vi "Self Event.vi"(9 "Priority?":bool, 10 "Msg Strategy":refnum<class "Msg Strategy.lvclass">, 11 "Base Event in":refnum<class "Base Event.lvclass">) -> (3 "Base Event out":refnum<class "Base Event.lvclass">)   [LabVIEW 2021, in "jettl.lvlib" / "Base Event.lvlib" / "Base Event.lvclass"]
uses:
  Base Event.lvclass
  Msg Strategy/Msg Strategy.lvclass
  Base Event.lvclass/Base Event.ctl
  Self Event/Self Event.lvlib
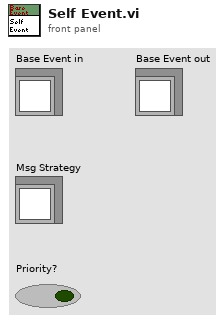
[diagram p1: front panel]
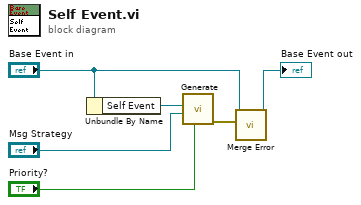
[diagram p0: block diagram]
diagram:
  n1 = Unbundle By Name("Base Event in") -> ("Self Event"=w5:refnum<data-value>)
  n2 = call "Generate.vi"("Priority?"="Priority?", "Msg Strategy"="Msg Strategy", "Self Event"=w5) -> ("error out"=w6:errorcluster)  [unwired: 8 in]
  n3 = call-dynamic "Merge Error.vi"("Error"=w6, "Base Event in"="Base Event in") -> ("Base Event out"=→"Base Event out":refnum<class "Base Event.lvclass">)  [unwired: 9 in]
